vi "FFT_based_oldcode.vi"() -> ()   [LabVIEW 2020]
uses:
  <vilib>/Utility/file.llb/Read Delimited Spreadsheet (DBL).vi
panel:
  out "Computational time (ticks)":u32
  out "Computational time":u32
  out "truth vs prediction":dbl[][](graph)
  out "Spectrum plot":cluster{i32, dbl, "spectrum out":dbl[]}(graph)
  out "Frequency Interval: delta(f)":dbl
  out "xf (frequency)":dbl[](array[numeric])
  out "size(s) 3":i32
  out "df (Hz) 3":dbl
  out "ploted signal from each selected frequency":dbl[][](graph)
  out "Input vs prediction":dbl[][](graph)
  out "truth vs prediction vs error":dbl[][](graph)
  out "Input vs prediction (zoomed)":dbl[][](graph)
  out "Time vs Acceleration \n Input learning length)":cluster{dbl[], dbl[]}[](graph)
  out "array w/ subset deleted":dbl[][](array[numeric])
  out "time":dbl[](array[numeric])
  out "Acceleration":dbl[](array[numeric])
  out "Time vs Acceleration graph(whole data)":cluster{"all rows":dbl[], "all rows":dbl[]}(graph)
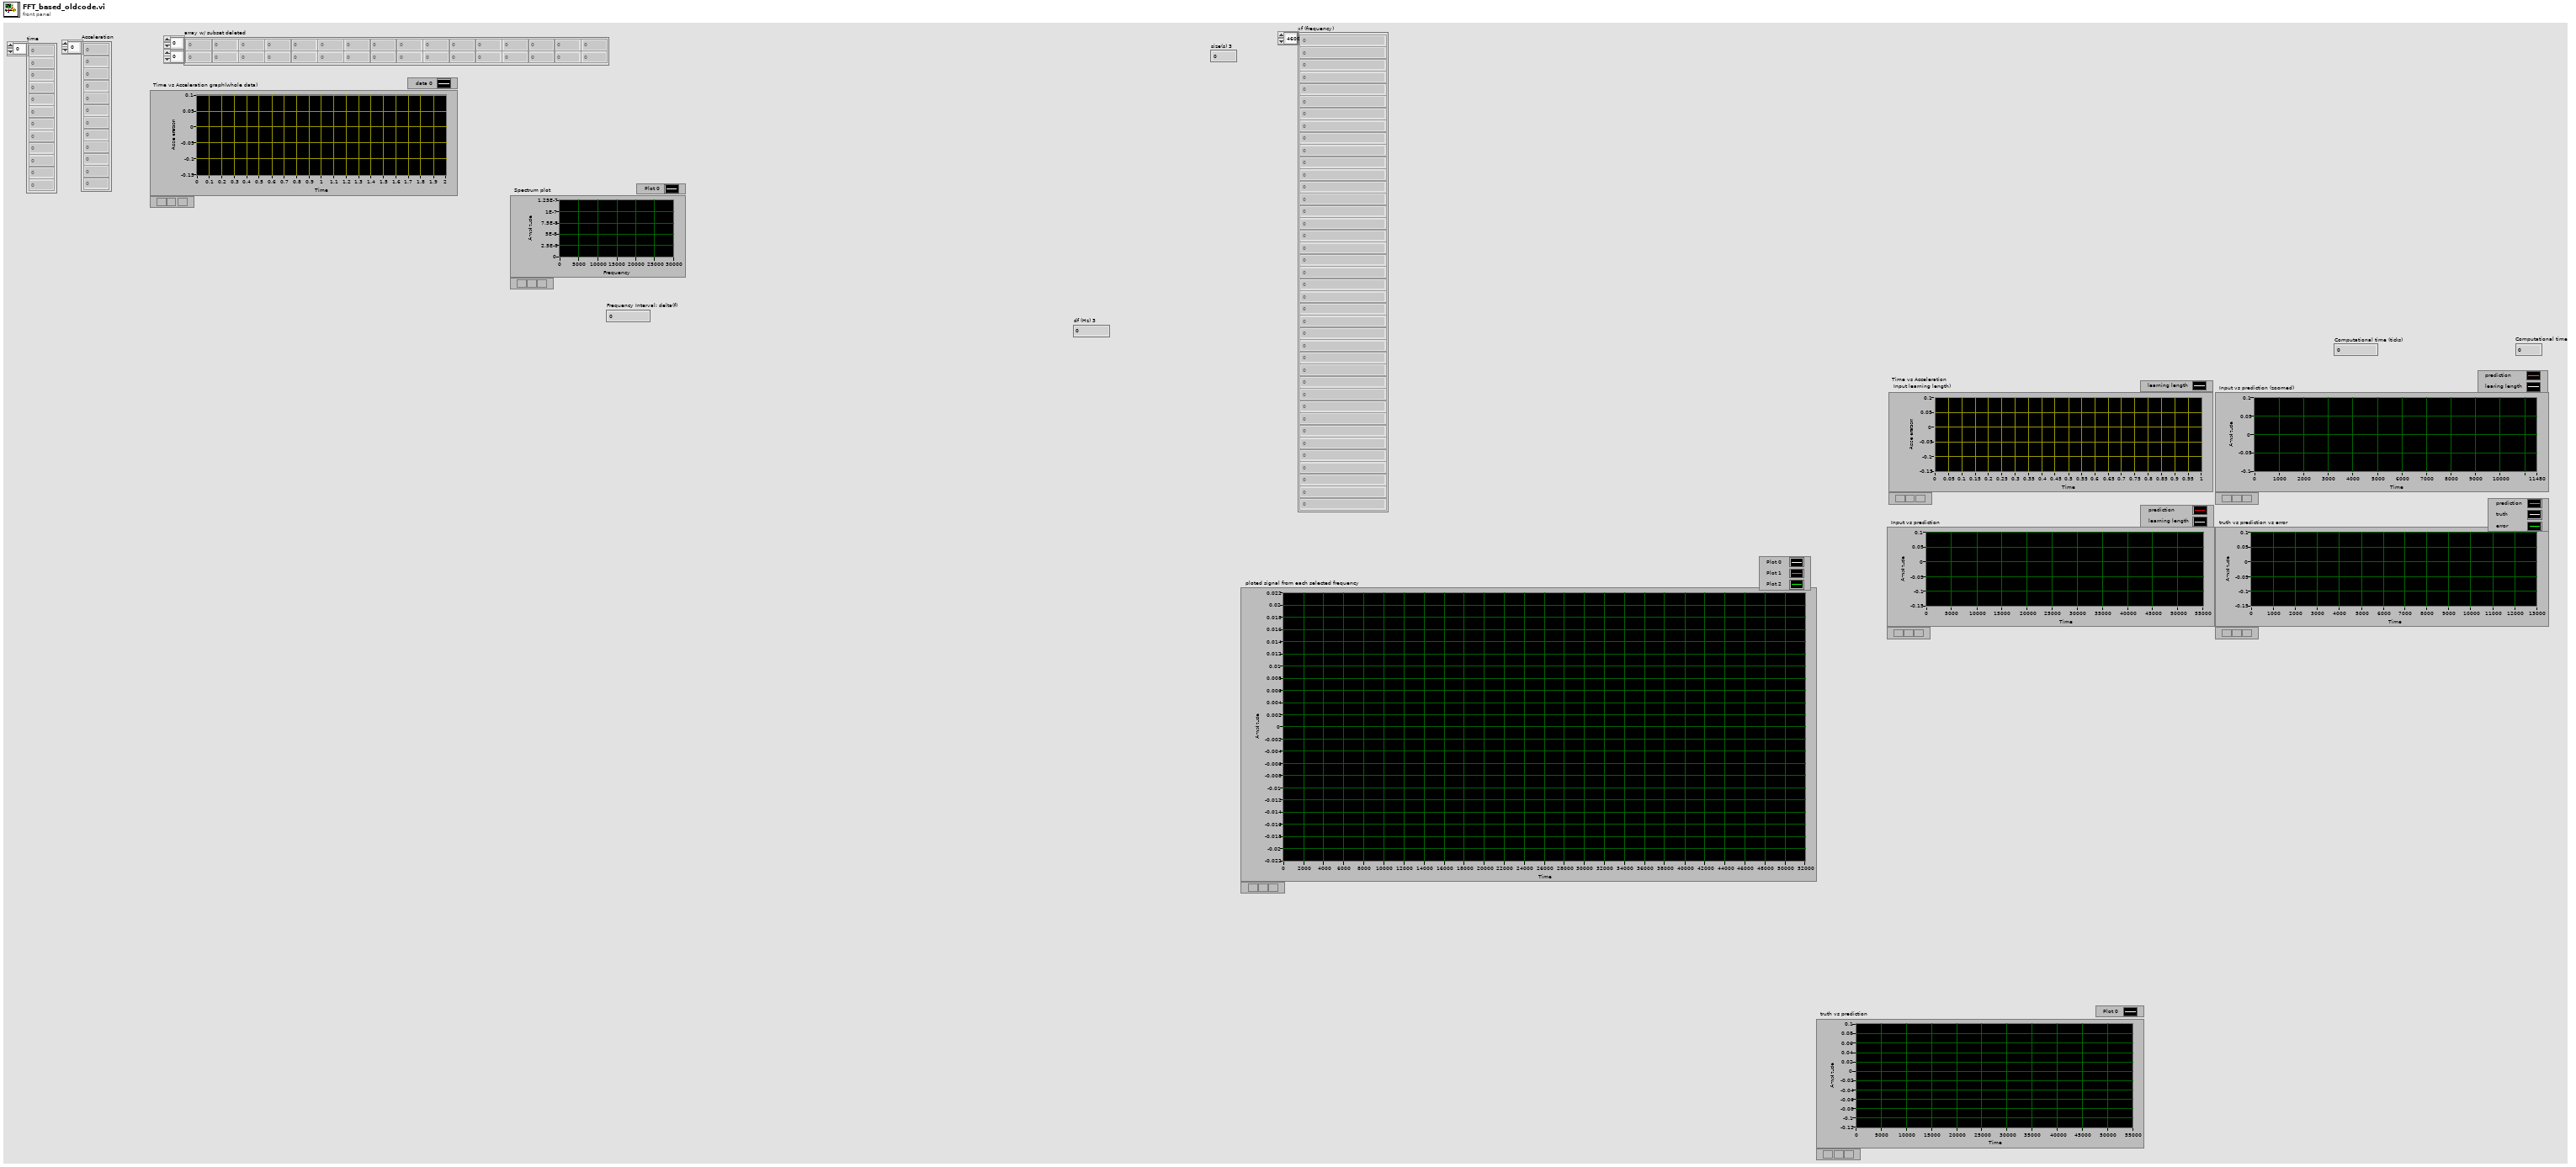
[diagram p1: front panel]
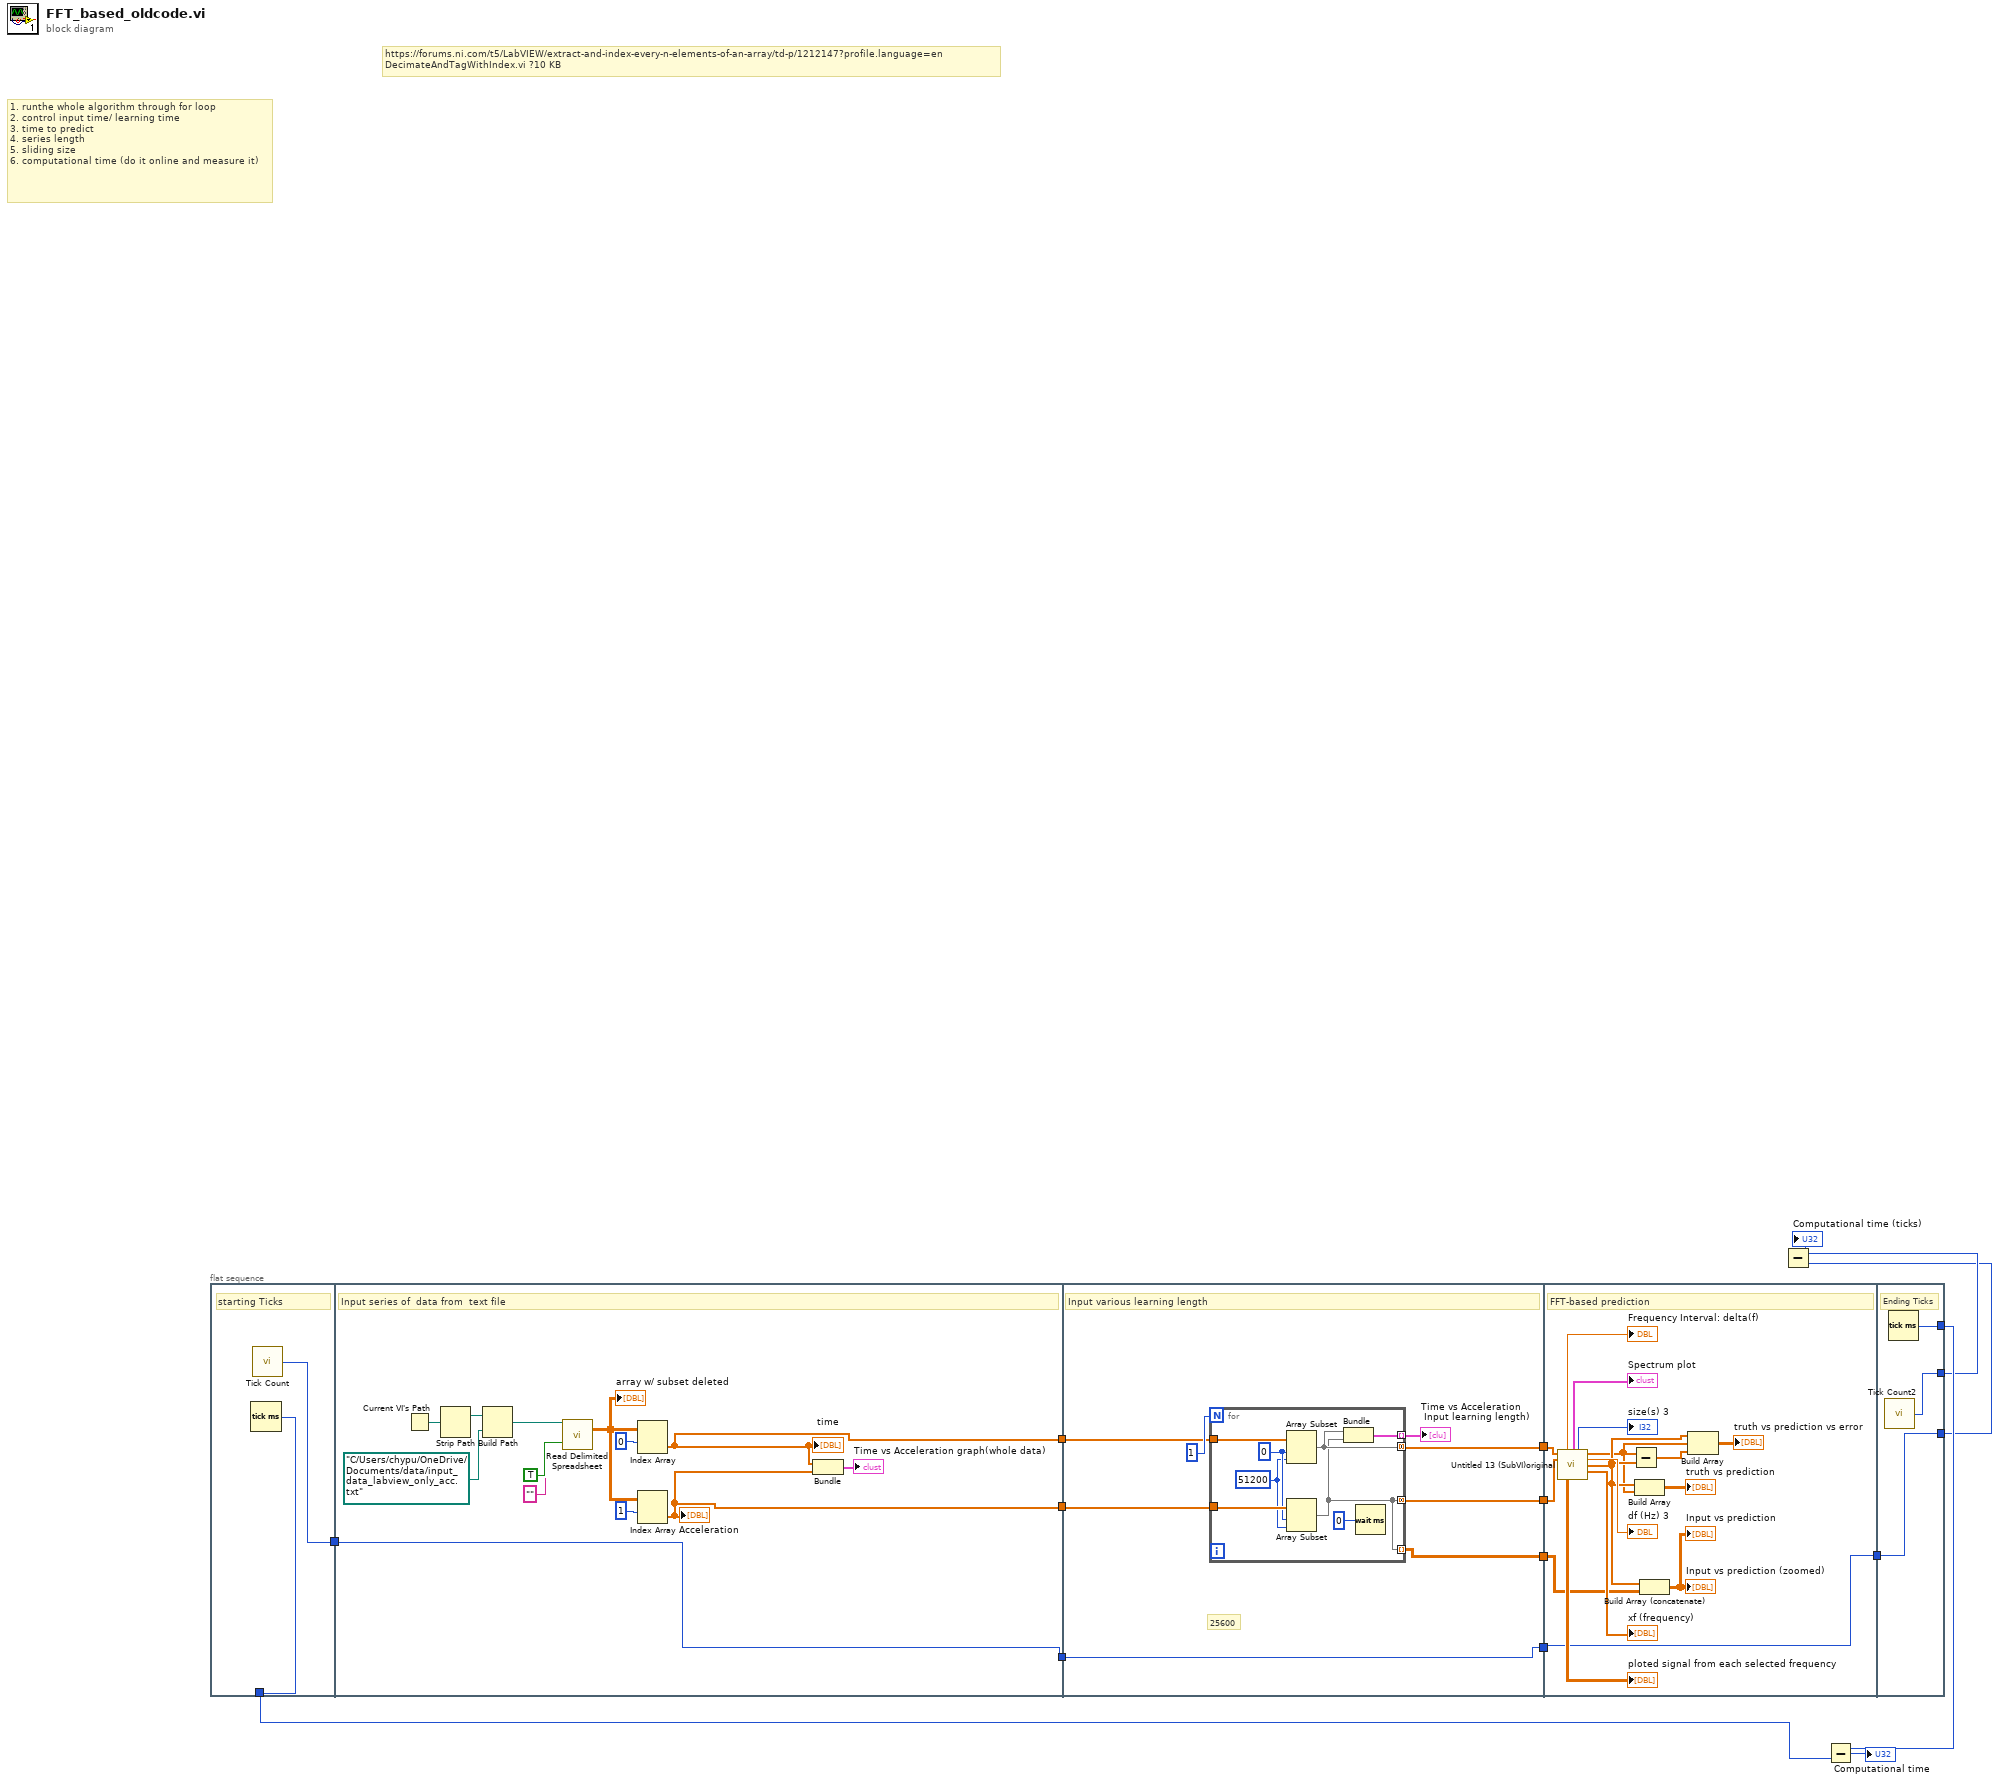
[diagram p0: block diagram]
diagram:
  # "1. runthe whole algorithm through for loop \n2. control input time/ learning time\n3. time to predict\n4. series length\n5. sliding size\n6. computational time (do it online and measure it)"
  # "https://forums.ni.com/t5/LabVIEW/extract-and-index-every-n-elements-of-an-array/td-p/1212147?profile.language=en\nDecimateAndTagWithIndex.vi ?10 KB"
  n1 = flat-sequence {
    tunnel: [w17] -> w4
    tunnel: [w16] -> w15
    tunnel: [w21] -> w14
    tunnel: [w20] -> w13
    tunnel: [w18] -> w12
    tunnel: w15 -> [w18]
    tunnel: w14 -> [w37]
    tunnel: w13 -> [w36]
    tunnel: [w34] -> w11
    tunnel: [w33] -> w10
    tunnel: [w32] -> w9
    tunnel: w12 -> [w31]
    tunnel: [w31] -> w8
    tunnel: w11 -> [w50]
    tunnel: w10 -> [w49]
    tunnel: w9 -> [w48]
    tunnel: w8 -> [w47]
    tunnel: [w47] -> w7
    tunnel: [w65] -> w6
    tunnel: [w64] -> w3
    tunnel: w7 -> [w63]
    tunnel: [w63] -> w2
    frame #0 {
      # "starting Ticks"
      n2 = Tick Count (ms)() -> (millisecond timer value=w17:u32)
      n3 = call "Tick Count"() -> ("Tick Count(uSec)"=w16:u32)
    }
    frame #1 {
      # "Input series of  data from  text file"
      n4 = Current VI's Path() -> (path=w28:path)
      n5 = Strip Path(path=w28) -> (stripped path=w29:path)  [unwired: 1 out]
      n6 = Build Path(base path=w29, name or relative path=path "C:/Users/chypu/OneDrive/Documents/data/input_data_labview_only_acc.txt") -> (appended path=w30:path)
      n7 = call-poly <vilib>:"Read Delimited Spreadsheet.vi"("file path (dialog if empty)"=w30, "transpose? (F)"=TRUE, "delimiter (\\t)"="" ("delimiter (\\t)")) -> ("all rows"=w27:dbl[][])  [unwired: 7 in, 5 out]
      "array w/ subset deleted" <- w27
      n8 = Index Array(array=w27, index (row)=0) -> (element=w21:dbl[])  [unwired: 1 in]
      "time" <- w21
      n9 = Index Array(array=w27, index (row)=1) -> (element=w20:dbl[])  [unwired: 1 in]
      "Acceleration" <- w20
      n10 = Bundle("all rows"=w21, "all rows"=w20) -> (→"Time vs Acceleration graph(whole data)":cluster{"all rows":dbl[], "all rows":dbl[]})  [unwired: 1 in]
    }
    frame #2 {
      # "25600"
      # "Input various learning length"
      n11 = for {
        N: 1 -> [_]
        tunnel: w37 -> [w46]
        tunnel: [w43] -> w34 mode=concatenating
        tunnel: w36 -> [w45]
        tunnel: [w41] -> w33 mode=concatenating
        tunnel: [w42] -> w35 mode=indexing
        tunnel: [w41] -> w32 mode=indexing
        w44 = 0
        w40 = 51200 ("length")
        n12 = Array Subset(array=w46, index=w44, length=w40) -> (w43:dbl[])
        n13 = Array Subset(array=w45, index=w44, length=w40) -> (w41:dbl[])
        n14 = Bundle(w43, w41) -> (w42:cluster{dbl[], dbl[]})  [unwired: 1 in]
        n15 = Wait (ms)(milliseconds to wait=u32 0) -> ()  [unwired: 1 out]
      }
      "Time vs Acceleration \n Input learning length)" <- w35
    }
    frame #3 {
      # "FFT-based prediction"
      n16 = call "Untitled 13 (SubVI)original.vi"("time"=w50, "acceleration"=w49) -> ("Frequency Interval: delta(f)"=→"Frequency Interval: delta(f)":dbl, "Spectrum plot"=→"Spectrum plot":cluster{i32, dbl, "spectrum out":dbl[]}, "size(s)"=→"size(s) 3":i32, "all rows"=w54:dbl[], "df (Hz)"=→"df (Hz) 3":dbl, "Array"=w55:dbl[], "xf (frequency)"=→"xf (frequency)":dbl[], "ploted signal from each selected frequency"=→"ploted signal from each selected frequency":dbl[][])  [unwired: 4 in, 2 out]
      n17 = Subtract(x=w54, y=w55) -> (x-y=w53:dbl[])
      n18 = Build Array(w55, w54) -> (→"truth vs prediction":dbl[][])
      n19 = Build Array (concatenate)(w55, w48) -> (→"Input vs prediction" →"Input vs prediction (zoomed)":dbl[][])
      n20 = Build Array(w55, w54, w53) -> (→"truth vs prediction vs error":dbl[][])
    }
    frame #4 {
      # "Ending Ticks"
      n21 = call "Tick Count2"() -> ("Tick Count(uSec)"=w64:u32)
      n22 = Tick Count (ms)() -> (millisecond timer value=w65:u32)
    }
  }
  n23 = Subtract(x=w3, y=w2) -> (x-y=→"Computational time (ticks)":u32)
  n24 = Subtract(x=w6, y=w4) -> (x-y=→"Computational time":u32)
